vi "RT Driver VI.vi"(6 "Device Clock":string, 9 "Device Inputs FIFO":refnum<k33>, 10 "Device Outputs FIFO":refnum<k33>, 11 "Device Reference":T1 format="%.0x") -> ()   [LabVIEW 2015, in "NI 9759 RevB Custom Device.lvlib"]
uses:
  NI 9759 RevB Custom Device.lvlib
  <vilib>/NI Veristand/Custom Device API/Custom Device Item Ref.ctl
  <vilib>/Platform/TimedLoop/XDataNode/timing_clust.ctl
  <vilib>/Platform/TimedLoop/XDataNode/nitl_modes.ctl
  <vilib>/Platform/TimedLoop/XDataNode/wakeup.ctl
  <vilib>/Platform/TimedLoop/XDataNode/XDataNode.xnode
  <vilib>/NI Veristand/Custom Device Tools/Custom Device Utility Library/Custom Device Utility Library.lvlib
  <vilib>/Platform/TimedLoop/XDataNode/XDNodeRunTimeDep.lvlib
  <vilib>/NI VeriStand/Custom Device API/Custom Device API.lvlib
panel:
  in  "Initialization Status Notifier":refnum<notifier>
  in  "Status Notifier":refnum<notifier>
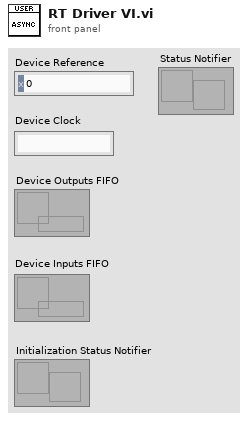
[diagram p1: front panel]
types:
  T1 = typedef "Custom Device API.lvlib/Custom Device Item Ref.ctl" = u64
  T2 = typedef "NI 9759 RevB Custom Device.lvlib/RT Data.ctl" = cluster{"Compiled Data":T3, "Device Inputs":dbl[], "Device Outputs":dbl[], "FPGA Refs":T7}
  T3 = typedef "NI 9759 RevB Custom Device.lvlib/Compiled Data.ctl" = cluster{"DeviceOutFIFO":refnum<k33>, "DeviceInFIFO":refnum<k33>, "Init":T4, "Status":T5, "9759 RevB":T6}
  T4 = typedef "NI 9759 RevB Custom Device.lvlib/RT Init Data.ctl" = cluster{"CPU":i32, "RIO Address":string, "Decimation":i32, "Priority":i32, "Name":string, "Bitfile Path":path, "Input FIFO Size":i32, "Output FIFO Size":i32, "Compile Time":dbl}
  T5 = typedef "NI 9759 RevB Custom Device.lvlib/RT Status.ctl" = cluster{"FIFO indexes":cluster{"code":i32, "loop duration":i32, "late count":i32}}
  T6 = typedef "NI 9759 RevB Custom Device.lvlib/9759 RevB.ctl" = cluster{"FIFO Indexes":cluster{"Read":cluster{"TP1":i32, "TP2":i32, "Analog1":i32, "Analog2":i32, "ISense1":i32, "ISense2":i32, "Battery":i32, "Temperature":i32, "ModulePresent":i32, "Fault1":i32, "Fault2":i32}, "Write":cluster{"ModuleEnable":i32, "ControlEnable1":i32, "ControlEnable2":i32, "Setpoint1":i32, "Setpoint2":i32}}, "Settings":cluster{"PositionCals":cluster{"TPArray (V)":sgl[], "TPArray (deg)":sgl[]}[], "ControlCals":cluster{"TLead (sec)":sgl, "TLag (sec)":sgl, "KRpos (V/deg)":sgl, "TIpos (sec)":sgl, "TDpos (sec)":sgl, "KRneg (V/deg)":sgl, "TIneg (sec)":sgl, "TDneg (sec)":sgl, "ThetaLHErrThresh (deg)":sgl, "ULH (V)":sgl, "ULHLag (sec)":sgl, "US (V)":sgl, "USLag (sec)":sgl, "ThetaLH (deg)":sgl, "MotorResistance (Ohms)":sgl, "BattNom (V)":sgl, "BattCompEnable":bool}[]}}
  T7 = typedef "NI 9759 RevB Custom Device.lvlib/FPGA Refs.ctl" = cluster{"Generic FPGA Ref":T8, "9759 RevB FPGA Ref":T9}
  T8 = typedef "NI 9759 RevB Custom Device.lvlib/Generic FPGA Ref.ctl" = refnum<k20>
  T9 = typedef "NI 9759 RevB Custom Device.lvlib/9759 RevB FPGA Ref.ctl" = refnum<k20>
  T10 = typedef "XDNodeRunTimeDep.lvlib/timing_clust.ctl" = cluster{"Expected End [f-1]":u64, "Actual End [f-1]":u64, "Finished Late? [f-1]":bool, "Expected End [i-1]":u64, "Actual End [i-1]":u64, "Finished Late? [i-1]":bool, "Expected Start [i]":u64, "Actual Start [i]":u64, "Expected Start [f]":u64, "Actual Start [f]":u64, "Source Name":string, "Structure Name":string, "Period":i64, "Deadline":i64, "Offset":i64, "Start":i64, "Priority":i32, "Timeout":i32, "Mode":T11, "Wakeup Reason":T12, "Error":errorcluster, "Source Type":string, "Secondary Source Type":string, "Global End Time":u64, "Global Start Time":u64, "Frame Duration":u64, "Iteration Duration":u64, "Assigned CPU":i32, "I/O Scan Engine Mode":u32}
  T11 = typedef "XDNodeRunTimeDep.lvlib/nitl_modes.ctl" = enum32{"No Change", "Process missed periods, maintain original phase", "Discard missed periods, maintain original phase", "Process missed periods, ignore original phase", "Discard missed periods, ignore original phase"}
  T12 = typedef "XDNodeRunTimeDep.lvlib/wakeup.ctl" = enum32{"Normal", "Aborted", "Asynchronous wakeup", "Timing source error", "Timed loop error", "Timeout"}
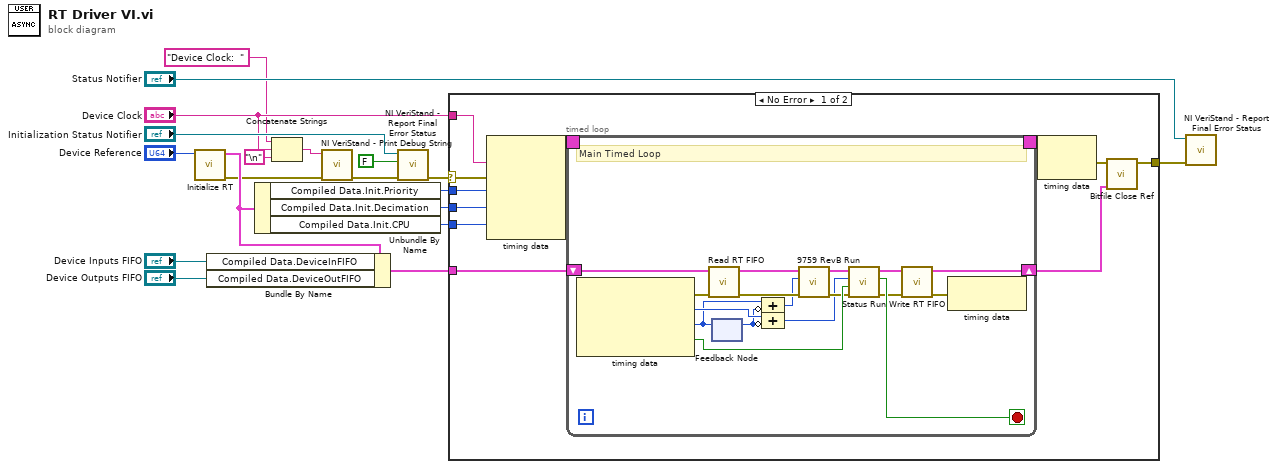
[diagram p0: block diagram]
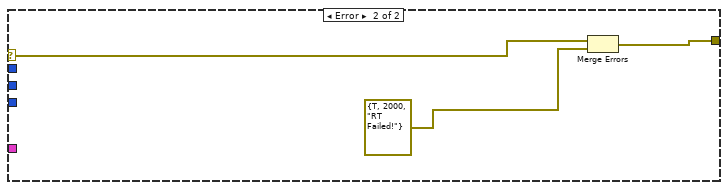
[diagram p2: hidden frame]
diagram:
  n1 = call "Initialize RT.vi"("Device Reference"="Device Reference") -> ("error out"=w6:errorcluster, "RT Data"=w7:T2)  [unwired: 9 in]
  n2 = Bundle By Name(cluster=w7, "Compiled Data.DeviceInFIFO"="Device Inputs FIFO", "Compiled Data.DeviceOutFIFO"="Device Outputs FIFO") -> (w11:T2)
  n3 = Unbundle By Name(w7) -> ("Compiled Data.Init.Priority"=w13:i32, "Compiled Data.Init.Decimation"=w14:i32, "Compiled Data.Init.CPU"=w12:i32)
  n4 = Concatenate Strings("Device Clock:  " ("string"), "Device Clock", "\n" ("string")) -> (w3:string)
  n5 = call <vilib>:"NI VeriStand - Print Debug String.vi"("error in (no error)"=w6, "Message"=w3) -> ("error out"=w5:errorcluster)  [unwired: 9 in]
  n6 = call <vilib>:"NI VeriStand - Report Final Error Status.vi"("error in (no error)"=w5, "Filter FIFO & Shutdown Errors (T)"=FALSE ("Filter FIFO Errors (T)"), "Status Notifier"="Initialization Status Notifier") -> ("error out"=w17:errorcluster)  [unwired: 8 out]
  n7 = case shown="No Error" w17 {
    selector: w17 -> [w28 w67]
    tunnel: "Device Clock" -> [w27 _]
    tunnel: [w20 w66] -> w10
    tunnel: w14 -> [w26 _]
    tunnel: w13 -> [w25 _]
    tunnel: w12 -> [w24 _]
    tunnel: w11 -> [w21 _]
    frame No Error {
      n8 = node-c288(w27, w28, w25, w26, w24) -> (w30:T10)
      n9 = timed-loop {
        timing: w30 -> [_]
        timing-out: [_] -> w29
        shift-right: [w45] -> w22
        shift-left: w21 -> [w41]
        stop <- w47 stop-if-true
        # "Main Timed Loop"
        n10 = node-c288() -> (w42:errorcluster, w40:i64, w32:i64, w39:bool)  [unwired: 1 in]
        n11 = call "Read RT FIFO.vi"("error in"=w42, "RT Data In"=w41) -> ("error out"=w36:errorcluster, "RT Data Out"=w38:T2)  [unwired: 8 in]
        n12 = feedback #1() -> (w33:i64)  [unwired: 1 in]
        n13 = feedback-in #1(w32) -> ()
        n14 = Compound Arithmetic op=ADD(w32, invert w33) -> (w31:i64)
        n15 = Compound Arithmetic op=ADD(w40, invert w33) -> (w34:i64)
        n16 = call "9759 RevB Run.vi"("error in"=w36, "Period (ns)"=w31, "RT Data In"=w38) -> ("error out"=w35:errorcluster, "RT Data Out"=w37:T2)  [unwired: 7 in]
        n17 = call "Status Run.vi"("error in"=w35, "Finished Late? [i-1]"=w39, "Iteration Duration"=w34, "RT Data In"=w37) -> ("error out"=w44:errorcluster, "Stop"=w47:bool, "RT Data Out"=w46:T2)  [unwired: 5 in]
        n18 = call "Write RT FIFO.vi"("error in"=w44, "RT Data In"=w46) -> ("error out"=w43:errorcluster, "RT Data Out"=w45:T2)  [unwired: 8 in]
        n19 = node-c288(w43) -> ()  [unwired: 1 out]
      }
      n20 = node-c288(w29) -> (w23:errorcluster)
      n21 = call "Bitfile Close Ref.vi"("RT Data In"=w22, "error in"=w23) -> ("error out"=w20:errorcluster)  [unwired: 9 in]
    }
    frame Error {
      n22 = Merge Errors(w67, errorcluster {"status"=TRUE, "code"=2000, "source"="RT Failed!"} ("error in")) -> (w66:errorcluster)
    }
  }
  n23 = call <vilib>:"NI VeriStand - Report Final Error Status.vi"("error in (no error)"=w10, "Status Notifier"="Status Notifier") -> ()  [unwired: 1 in, 9 out]
